vi "Drive Controller.vi"(8 "error in":errorcluster) -> ()   [LabVIEW 2020]
doc: "This VI executes continuously carrying out the current operation and responding to updates or new operation requests. It will often contain the timing or control code that is difficult to place directly in TeleOp. This VI generally opens all sensors and motors and isolates the rest of the robot code from knowing implementation details of how the operations are carried out."
uses:
  <vilib>/Rock Robotics/WPI/Framework/Completion Status.ctl
  Drive Setpoints.ctl
  Drive Operations.ctl
  <vilib>/Rock Robotics/WPI/ThirdParty/Phoenix-LabVIEW/Motor Controller/Controls/CTRE_Phoenix_MotorControl_ControlMode.ctl
panel:
  in  "Interactive Values":T1
  in  "Buttons":cluster{"Execute Cmd":bool, "Abort Cmd":bool}
  out "Command Timing":cluster{"Start Time (ms)":u32, "Iterations":i32}
  out "Status":T3
  out "Setpoints":T4(graph)
  out "Current\nCmd":string
  # "Tip: The graph shows the motor setpoints. It may also be helpful to observe inputs and sensor values.\nYou may also want to display tuning or debugging controls."
  # "Interactive Command: You may fill in the settings for a command\nand schedule it with the Execute button. You can observe and abort\nany command while fine tuning the code for the controller."
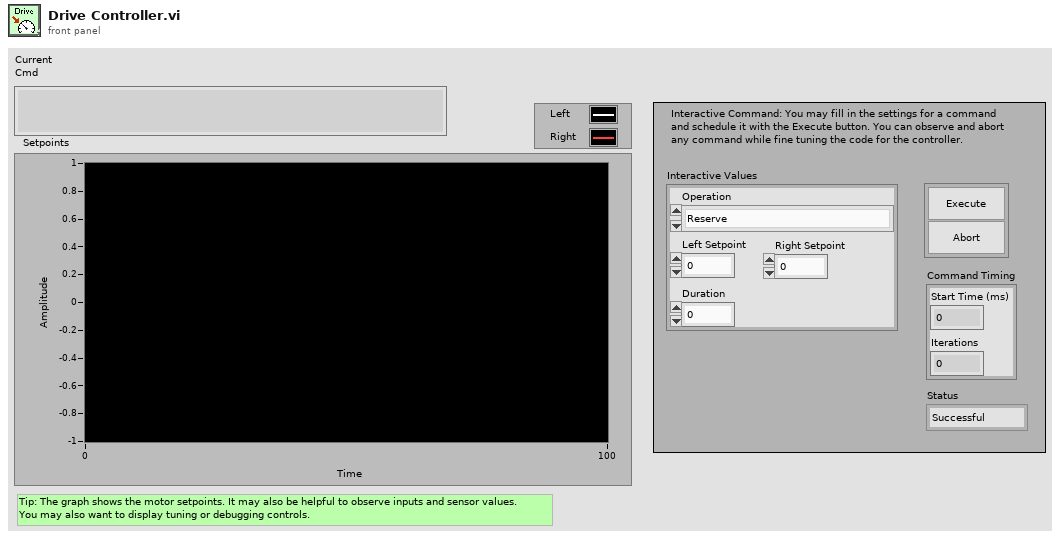
[diagram p1: front panel]
types:
  T1 = typedef "Drive Setpoints.ctl" = cluster{"Operation":T2, "Left Setpoint":dbl, "Right Setpoint":dbl, "Duration":dbl}
  T2 = typedef "Drive Operations.ctl" = enum16{"Reserve", "Read Current", "Immediate", "Drive for Time", "Drive for Distance"}
  T3 = typedef "Completion Status.ctl" = enum16{"Successful", "Aborted", "Incomplete"}
  T4 = cluster{"Left Setpoint":dbl, "Right Setpoint":dbl}
  T5 = typedef "WPI_MotorControlDeviceRef.ctl" = cluster{"DeviceStatus":errorcluster, "Type":T6, "PWM":cluster{"PWM Channel":T7, "DeadBand":T8}, "CAN":cluster{"Device Number":u8, "SetOutput VI Ref":variant, "GetOutput VI Ref":variant, "Enable VI Ref":variant, "Disable VI Ref":variant, "Data":variant}, "Invert":bool, "DIO PWM":cluster{"PWM \"Enable\" Channel":T7, "DIOChannel":T9, "PWM Rate":dbl}}
  T6 = typedef "WPI_MotorControlType.ctl" = enum16{"PWM", "CAN", "DIO PWM"}
  T7 = typedef "FPGA_DIOPWMChannel.ctl" = enum8{"PWM 0", "PWM 1", "PWM 2", "PWM 3", "PWM 4", "PWM 5", "PWM 6", "PWM 7", "PWM 8", "PWM 9", "PWM MXP 0", "PWM MXP 1", "PWM MXP 2", "PWM MXP 3", "PWM MXP 4", "PWM MXP 5", "PWM MXP 6", "PWM MXP 7", "PWM MXP 8", "PWM MXP 9", "Invalid"}
  T8 = typedef "WPI_PWMDeadband.ctl" = cluster{"Name":string, "maxPositivePwm":i32, "minPositivePwm":i32, "centerPwm":i32, "maxNegativePwm":i32, "minNegativePwm":i32, "angularRange":u16}
  T9 = typedef "FPGA_DIOChannel.ctl" = enum8{"DIO 0", "DIO 1", "DIO 2", "DIO 3", "DIO 4", "DIO 5", "DIO 6", "DIO 7", "DIO 8", "DIO 9", "DIO MXP 0", "DIO MXP 1", "DIO MXP 2", "DIO MXP 3", "DIO MXP 4", "DIO MXP 5", "DIO MXP 6", "DIO MXP 7", "DIO MXP 8", "DIO MXP 9", "DIO MXP 10", "DIO MXP 11", "DIO MXP 12", "DIO MXP 13", "DIO MXP 14", "DIO MXP 15", "SPI Port CS1", "SPI Port CS2", "SPI Port CS3", "SPI Port MISO", "SPI Port MOSI", "Invalid"}
  T10 = cluster{"PhoenixMotorControlDevRef":T5, "error out":errorcluster, "PhoenixMotorControlDevRef":T5, "error out":errorcluster}
  T11 = typedef "Command Status Info.ctl" = cluster{"Name":string, "Status":T3, "notifier out":T12}
  T12 = typedef "Completion Notifier.ctl" = refnum<notifier>
  T13 = cluster{"SubSystem Data":T1, cluster{"Start Time (ms)":u32, "Iterations":i32}, cluster{"Command Info":T11, "Description":string, "Default Command":T1, "queue out":refnum<queue>, "Subsystem Name":string}}
  T14 = typedef "CTRE_Phoenix_MotorControl_ControlMode.ctl" = u16
  T15 = cluster{"SubSystem Data":T1, cluster{"Start Time (ms)":u32, "Iterations":i32}, "Default Command Arguments":cluster{"Command Info":T11, "Description":string, "Default Command":T1, "queue out":refnum<queue>, "Subsystem Name":string}}
  T16 = cluster{"Don't move motors while reserved":dbl, "Don't move motors while reserved":dbl}
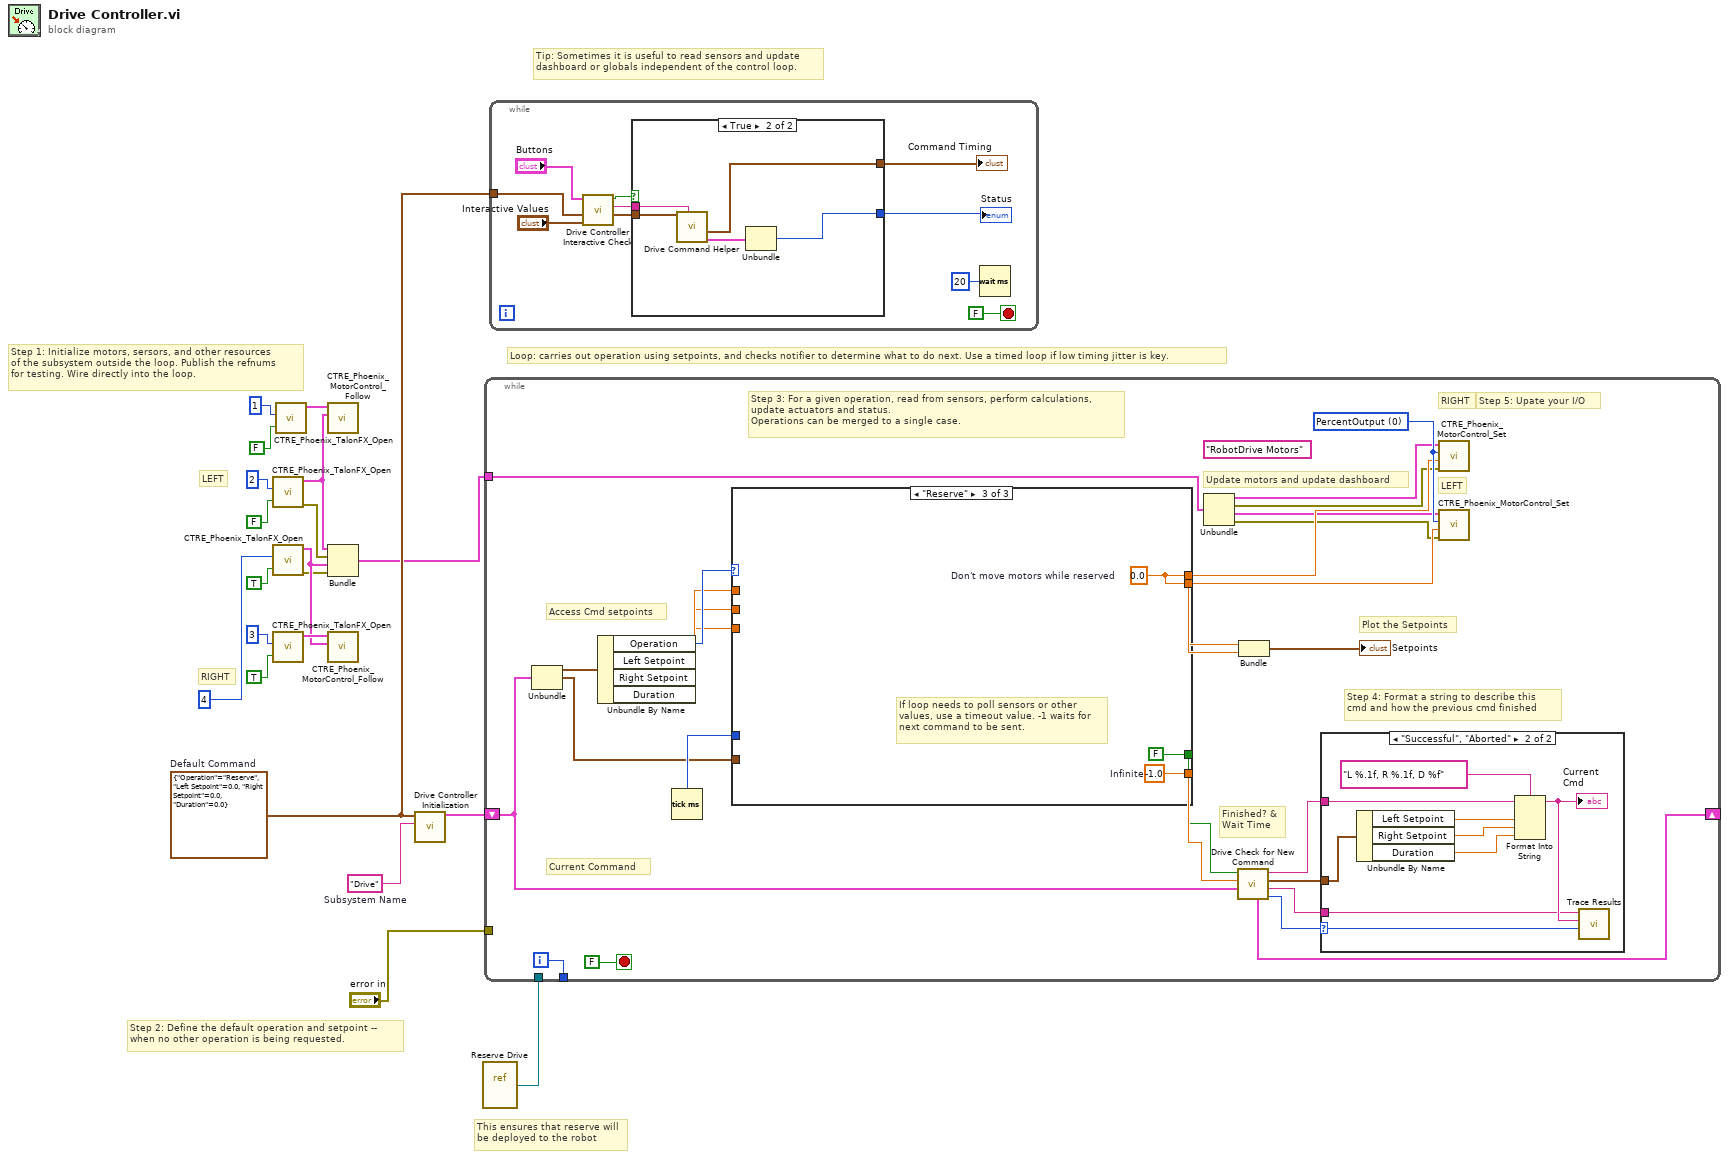
[diagram p0: block diagram]
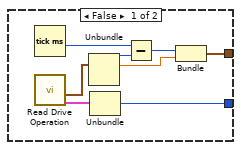
[diagram p2: hidden frame]
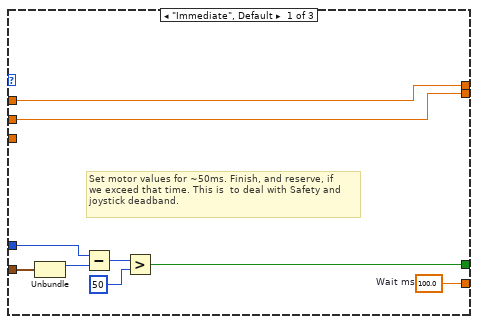
[diagram p4: hidden frame]
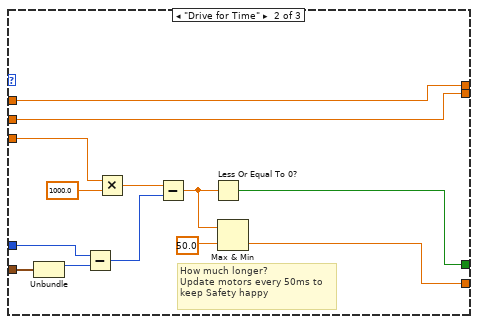
[diagram p5: hidden frame]
diagram:
  w16 = T1 {"Operation"=enum."Reserve", "Left Setpoint"=0.0, "Right Setpoint"=0.0, "Duration"=0.0}  # Default Command
  w20 = "Drive"  # Subsystem Name
  # "RIGHT"
  # "LEFT"
  # "This ensures that reserve will\nbe deployed to the robot"
  # "Tip: Sometimes it is useful to read sensors and update\ndashboard or globals independent of the control loop."
  # "Step 2: Define the default operation and setpoint --\nwhen no other operation is being requested."
  # "Step 1: Initialize motors, sersors, and other resources\nof the subsystem outside the loop. Publish the refnums\nfor testing. Wire directly into the loop."
  # "Loop: carries out operation using setpoints, and checks notifier to determine what to do next. Use a timed loop if low timing jitter is key."
  n1 = call <vilib>:"CTRE_Phoenix_TalonFX_Open.vi"("Invert"=FALSE, "Device Number"=u8 2) -> ("error out"=w4:errorcluster, "PhoenixMotorControlDevRef"=w5:T5)  [unwired: 8 in]
  n2 = call <vilib>:"CTRE_Phoenix_TalonFX_Open.vi"("Invert"=TRUE, "Device Number"=u8 4) -> ("error out"=w2:errorcluster, "PhoenixMotorControlDevRef"=w3:T5)  [unwired: 8 in]
  n3 = call <vilib>:"CTRE_Phoenix_TalonFX_Open.vi"("Invert"=TRUE, "Device Number"=u8 3) -> ("PhoenixMotorControlDevRef"=w10:T5)  [unwired: 8 in, 1 out]
  n4 = call <vilib>:"CTRE_Phoenix_TalonFX_Open.vi"("Invert"=FALSE, "Device Number"=u8 1) -> ("PhoenixMotorControlDevRef"=w15:T5)  [unwired: 8 in, 1 out]
  n5 = call <vilib>:"CTRE_Phoenix_MotorControl_Follow.vi"("Master Controller to Follow"=w5, "PhoenixMotorControlDevRef"=w15) -> ()  [unwired: 8 in, 2 out]
  n6 = Bundle("PhoenixMotorControlDevRef"=w5, "error out"=w4, "PhoenixMotorControlDevRef"=w3, "error out"=w2) -> (w1:T10)  [unwired: 1 in]
  n7 = call <vilib>:"CTRE_Phoenix_MotorControl_Follow.vi"("Master Controller to Follow"=w3, "PhoenixMotorControlDevRef"=w10) -> ()  [unwired: 8 in, 2 out]
  n8 = call "Drive Controller Initialization.vi"("Subsystem Name"=w20, "Default Command"=w16) -> ("Current Command"=w18:T13)  [unwired: 9 in]
  n9 = vi-ref "Reserve Drive.vi"() -> (w17:refnum<vi>)
  n10 = while {
    shift-right: [w36] -> _
    shift-left: w18 -> [w29]
    tunnel: [w45] -> _
    tunnel: "error in" -> [_]
    tunnel: w17 -> [_]
    tunnel: w1 -> [w25]
    i -> [w45]
    stop <- FALSE stop-if-true
    w28 = T14 0 items=["PercentOutput"=0, "Position"=1, "Velocity"=2, "Current"=3, "Follower"=5, "MotionProfile"=6, "MotionMagic"=7, "MotionProfileArc"=10, "Disabled"=15] ("Control Mode")
    (unwired) "RobotDrive Motors" ("Name")
    # "RIGHT"
    # "LEFT"
    # "Step 5: Upate your I/O"
    # "Step 4: Format a string to describe this\ncmd and how the previous cmd finished"
    # "Current Command"
    # "Update motors and update dashboard"
    # "Plot the Setpoints"
    # "Access Cmd setpoints"
    # "Finished? &\nWait Time"
    # "Step 3: For a given operation, read from sensors, perform calculations,\nupdate actuators and status.\nOperations can be merged to a single case."
    n11 = Unbundle(w29) -> ("SubSystem Data"=w43:T1, w30:cluster{"Start Time (ms)":u32, "Iterations":i32})  [unwired: 1 out]
    n12 = Unbundle By Name(w43) -> ("Operation"=w42:T2, "Left Setpoint"=w41:dbl, "Right Setpoint"=w40:dbl, "Duration"=w39:dbl)
    n13 = Tick Count (ms)() -> (millisecond timer value=w38:u32)
    n14 = case shown="\"Reserve\"" w42 {
      tunnel: [w64 w65 w80] -> w35
      tunnel: [w57 w72 FALSE ("ignore previous (F)")] -> w34
      tunnel: w30 -> [w56 w74 _]
      tunnel: [w63 w71 w78] -> w26
      tunnel: [w62 w70 w78] -> w27
      tunnel: w41 -> [w63 w71 _]
      tunnel: w40 -> [w62 w70 _]
      tunnel: w39 -> [_ w69 _]
      tunnel: w38 -> [w58 w68 _]
      frame "Immediate", Default {
        w64 = 100.0  # Wait ms
        # "Set motor values for ~50ms. Finish, and reserve, if\nwe exceed that time. This is  to deal with Safety and\njoystick deadband."
        n15 = Unbundle(w56) -> ("Start Time (ms)"=w59:u32)  [unwired: 1 out]
        n16 = Subtract(x=w58, y=w59) -> (x-y=w60:u32)
        n17 = Greater?(x=w60, y=u8 50 ("Left Motor")) -> (0:w57:bool)
      }
      frame "Drive for Time" {
        # "How much longer?\nUpdate motors every 50ms to\nkeep Safety happy"
        n18 = Unbundle(w74) -> ("Start Time (ms)"=w73:u32)  [unwired: 1 out]
        n19 = Subtract(x=w68, y=w73) -> (x-y=w77:u32)
        n20 = Multiply(x=w69, y=1000.0) -> (x*y=w76:dbl)
        n21 = Subtract(x=w76, y=w77) -> (x-y=w67:dbl)
        n22 = Less Or Equal To 0?(x=w67) -> (x <= 0?=w72:bool)
        n23 = Max & Min(x=w67, y=50.0) -> (min(x,y)=w65:dbl)  [unwired: 1 out]
      }
      frame "Reserve" {
        w78 = 0.0  # Don't move motors while reserved
        w80 = -1.0  # Infinite
        # "If loop needs to poll sensors or other\nvalues, use a timeout value. -1 waits for\nnext command to be sent."
      }
    }
    n24 = Unbundle(w25) -> ("PhoenixMotorControlDevRef"=w24:T5, "error out"=w23:errorcluster, "PhoenixMotorControlDevRef"=w22:T5, "error out"=w21:errorcluster)
    n25 = call "Drive Check for New Command.vi"("input cluster"=w29, "Wait time (ms)"=w35, "Finished?"=w34) -> ("Completion"=w37:T3, "Subsystem Name"=w31:string, "Current Command"=w32:T1, "Initial Trace String"=w33:string, "Next Command"=w36:T15)  [unwired: 4 in]
    n26 = Bundle("Don't move motors while reserved"=w26, "Don't move motors while reserved"=w27) -> (→"Setpoints":T16)  [unwired: 1 in]
    n27 = case shown="\"Successful\", \"Aborted\"" w37 {
      selector: w37 -> [_ w55]
      tunnel: w33 -> [_ w50]
      tunnel: w32 -> [_ w51]
      tunnel: w31 -> [_ w47]
      frame "Incomplete", Default {
        # "Continuing current command"
      }
      frame "Successful", "Aborted" {
        # "Report and setup for next command"
        n28 = Unbundle By Name(w51) -> ("Left Setpoint"=w53:dbl, "Right Setpoint"=w54:dbl, "Duration"=w48:dbl)
        n29 = Format Into String(format string="L %.1f, R %.1f, D %f", initial string=w50, w53, w54, w48) -> (resulting string=w49:string)  [unwired: 1 in, 1 out]
        "Current\nCmd" <- w49
        n30 = call <vilib>:"Trace Results.vi"("Status of previous command"=w55, "Description"=w49, "Subsystem"=w47) -> ()  [unwired: 9 in]
      }
    }
    n31 = call <vilib>:"CTRE_Phoenix_MotorControl_Set.vi"("error in (no error)"=w23, "Output"=w26, "Control Mode"=w28, "PhoenixMotorControlDevRef"=w24) -> ()  [unwired: 6 in, 2 out]
    n32 = call <vilib>:"CTRE_Phoenix_MotorControl_Set.vi"("error in (no error)"=w21, "Output"=w27, "Control Mode"=w28, "PhoenixMotorControlDevRef"=w22) -> ()  [unwired: 6 in, 2 out]
  }
  n33 = while {
    tunnel: w16 -> [w82]
    stop <- FALSE stop-if-true
    n34 = call "Drive Controller Interactive Check.vi"("Interactive Command In"="Interactive Values", "Default Command"=w82, "Buttons"="Buttons") -> ("Interactive Command Out"=w84:T1, "Trace String"=w85:string, "Schedule"=w86:bool)  [unwired: 6 in]
    n35 = case shown="True" w86 {
      tunnel: [w95 w103] -> w87
      tunnel: [w94 w99] -> w88
      tunnel: w85 -> [_ w101]
      tunnel: w84 -> [_ w100]
      frame False {
        n36 = Tick Count (ms)() -> (millisecond timer value=w98:u32)
        n37 = call "Read Drive Operation.vi"() -> ("Command Info"=w92:T11, "SubSystem Data"=w91:T1)  [unwired: 9 in, 1 out]
        n38 = Unbundle(w91) -> ("Operation"=w96:T2, "Left Setpoint"=w93:dbl)  [unwired: 2 out]
        n39 = Unbundle(w92) -> ("Status"=w95:T3)  [unwired: 2 out]
        n40 = Subtract(x=w98, y=w96) -> (x-y=w97:u32)
        n41 = Bundle(w97, "Left Setpoint"=w93) -> (w94:cluster{u32, "Left Setpoint":dbl})  [unwired: 1 in]
      }
      frame True {
        n42 = call "Drive Command Helper.vi"("Description"=w101, "SubSystem Data"=w100) -> ("Command Info Out"=w102:T11, "Command Timing"=w99:cluster{"Start Time (ms)":u32, "Iterations":i32})  [unwired: 7 in, 1 out]
        n43 = Unbundle(w102) -> ("Status"=w103:T3)  [unwired: 2 out]
      }
    }
    "Status" <- w87
    "Command Timing" <- w88
    n44 = Wait (ms)(milliseconds to wait=u32 20) -> ()  [unwired: 1 out]
  }
